vi "Convert Sensor Status to RGB value.vi"(9 "Sensor Healthy":bool, 10 "Sensor Enabled":bool, 11 "Sensor Present":bool) -> (3 "Sensor Status":u32(colorbox))   [LabVIEW 2014]
uses:
  Aircraft Information/Controls/Sensor Healthy.ctl
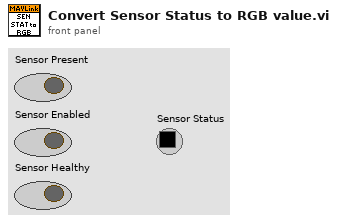
[diagram p1: front panel]
types:
  T1 = typedef "Sensor Healthy.ctl" = u32
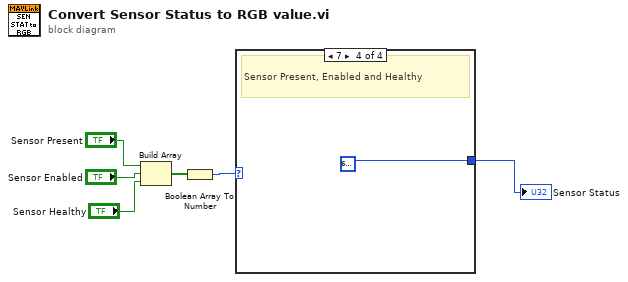
[diagram p0: block diagram]
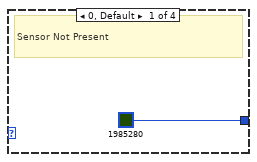
[diagram p2: hidden frame]
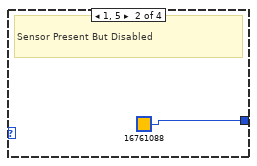
[diagram p3: hidden frame]
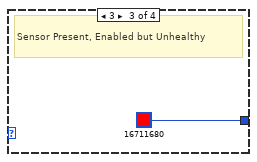
[diagram p4: hidden frame]
diagram:
  n1 = Build Array("Sensor Present", "Sensor Enabled", "Sensor Healthy") -> (w3:bool[])
  n2 = Boolean Array To Number(Boolean array=w3) -> (number=w2:u32)
  n3 = case shown="7" w2 {
    tunnel: [u32 1985280 u32 16761088 u32 16711680 T1 6618880 ("Color Box")] -> w1
    frame 0, Default {
      # "Sensor Not Present"
    }
    frame 1, 5 {
      # "Sensor Present But Disabled"
    }
    frame 3 {
      # "Sensor Present, Enabled but Unhealthy"
    }
    frame 7 {
      # "Sensor Present, Enabled and Healthy"
    }
  }
  "Sensor Status" <- w1
